vi "MIDI reader.vi"(8 "error in":errorcluster) -> (0 "error out":errorcluster, 2 "Note Events":T1[](array[typedef]), 3 "Array":T2(array[cluster]) {"U8" format="%x"; "Bytes" format="%02d"; "U8" format="%x"})   [LabVIEW 2016]
uses:
  Notes.ctl
  Midi data.ctl
panel:
  out "Time Sig Denom":u8
  out "data":u8[](array[numeric]) format="%x"
  out "Sequencer Event":string
  out "Device Name":string
  out "Program Name":string
  out "Cue Point":string
  out "Marker":string
  out "Lyric":string
  out "Instr Name":string
  out "CopyRight":string
  out "Text":string
  out "Track Name":string
  out "Key Signature":i8[](array[numeric])
  out "Time Sig":u8[](array[numeric])
  out "SMPTE Offset":u8[](array[numeric])
  out "MIDI Port":u8
  out "MIDI Channel":u8
  out "MIDI cue":u16
  out "size(s)":i32[](array[numeric])
  out "ms/b":u32
  out "Track length":u32
  out "Division":u16
  out "Number of tracks":u16
  out "Format":u16
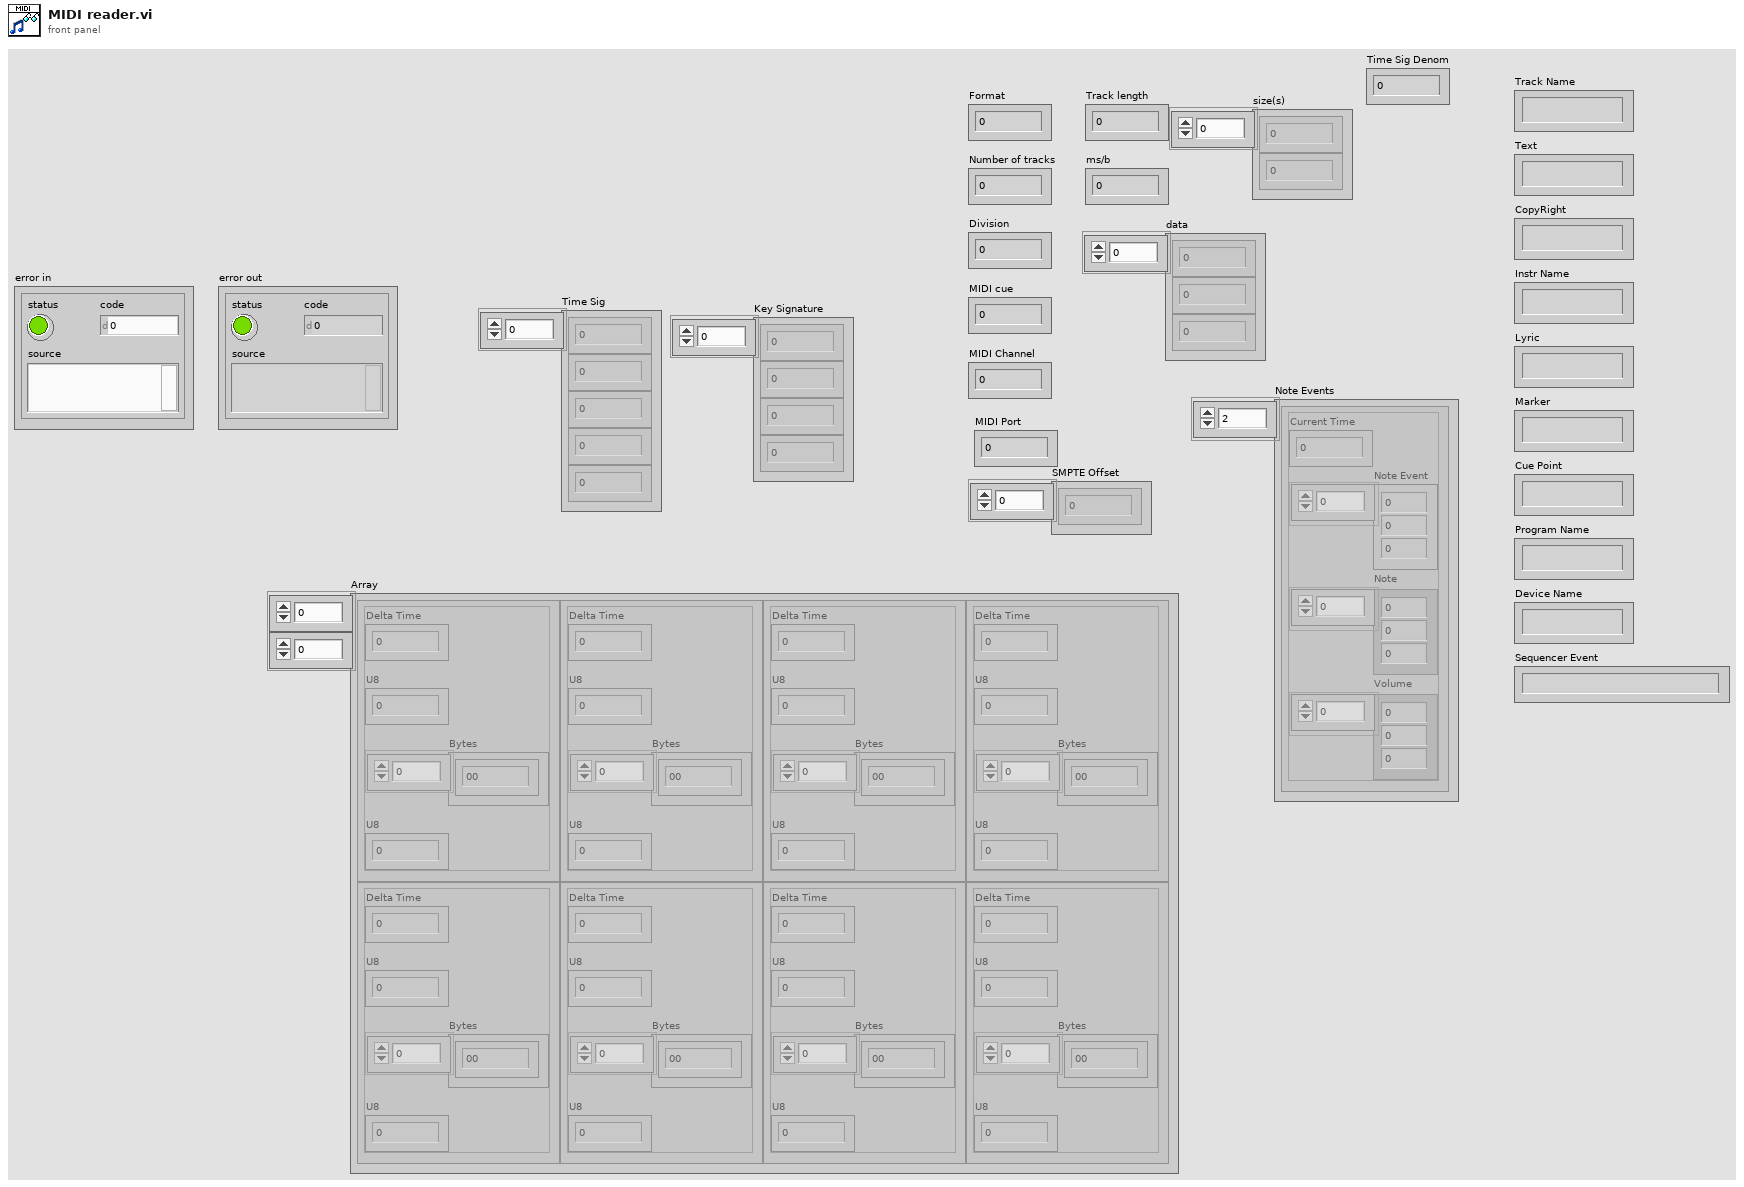
[diagram p1: front panel]
types:
  T1 = typedef "Notes.ctl" = cluster{"Current Time":u32, "Note Event":u32[], "Note":u32[], "Volume":u32[]}
  T2 = cluster{"Delta Time":u32, "U8":u8, "Bytes":u32[], "U8":u8}[][]
  T3 = enum16{"big-endian, network order", "native, host order", "little-endian"}
  T4 = cluster{"Delta Time":u32, "U8":u8, "Bytes":u32[], "U8":u8}[]
  T5 = typedef "Midi data.ctl" = cluster{"Delta Time":u32, "Event Status":u8, "Bytes":u32[], "Event Val":u8}
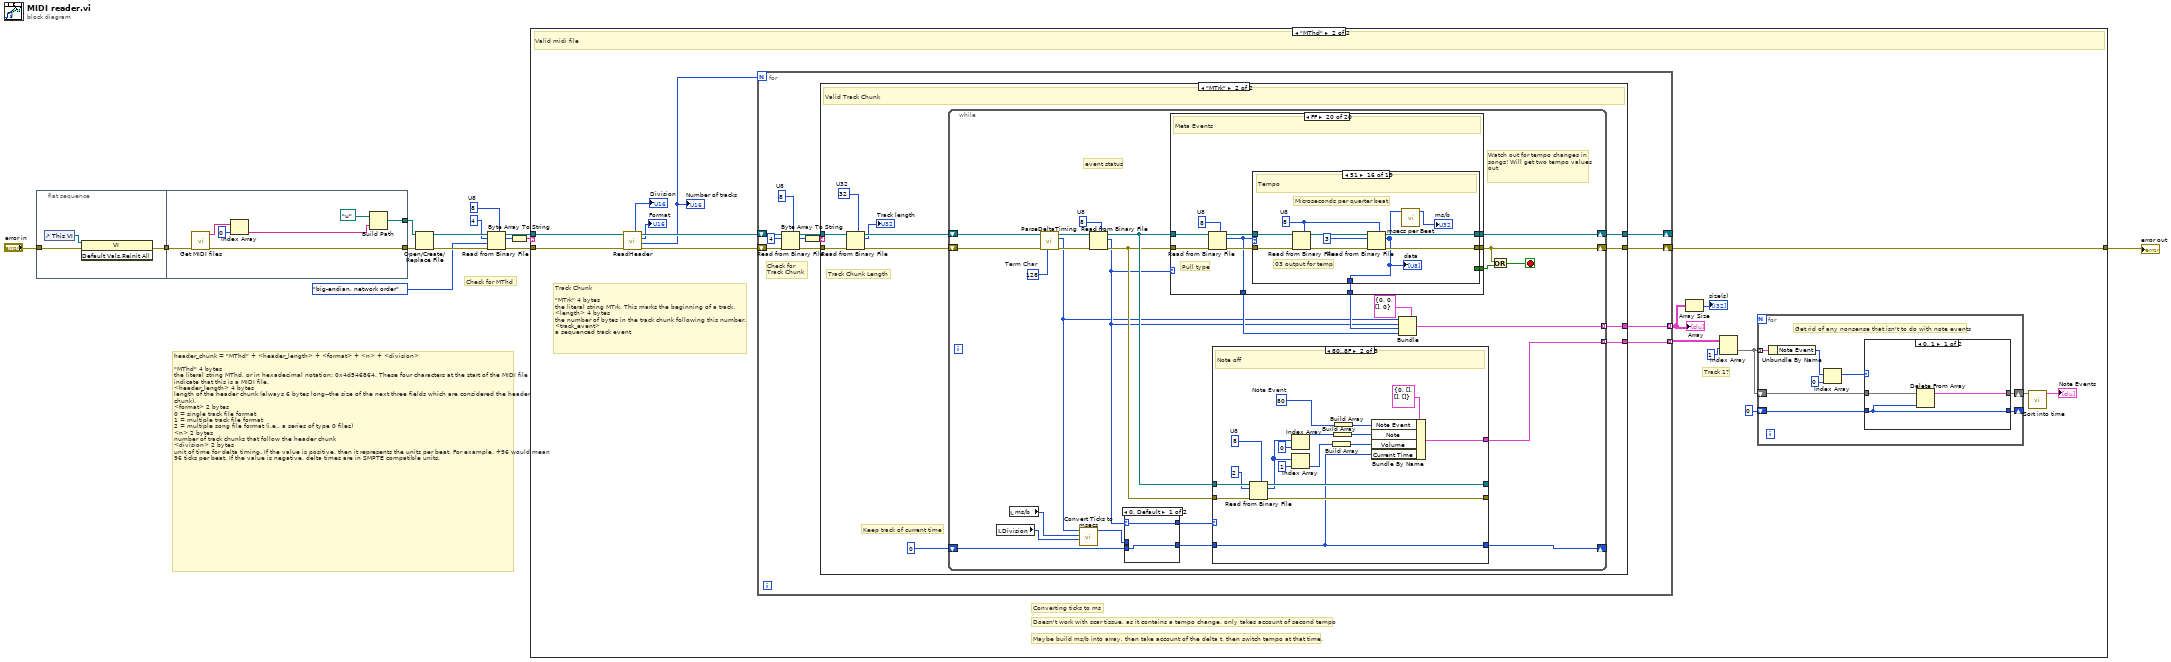
[diagram p0: block diagram]
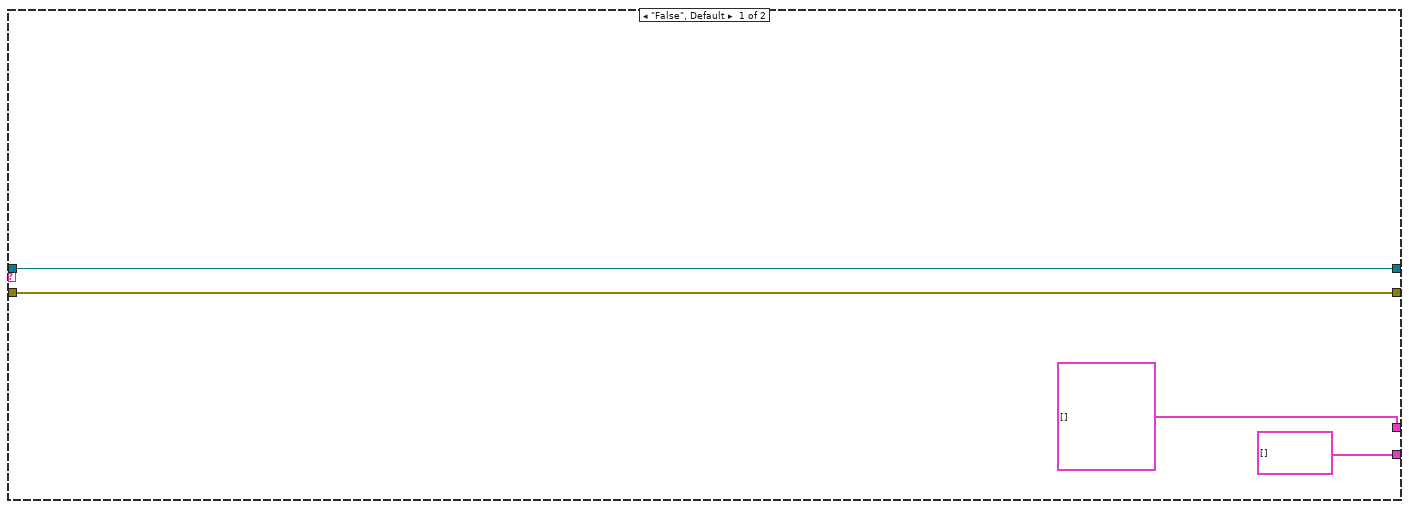
[diagram p3: hidden frame]
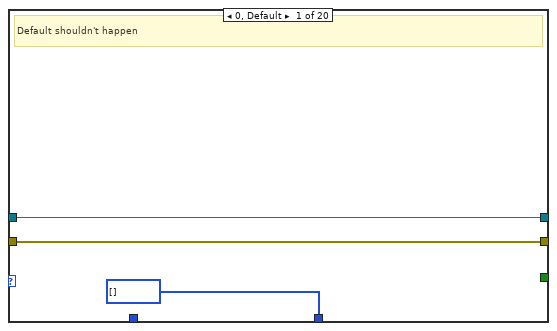
[diagram p4: hidden frame]
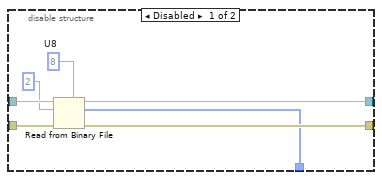
[diagram p6: hidden frame]
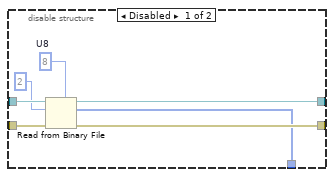
[diagram p8: hidden frame]
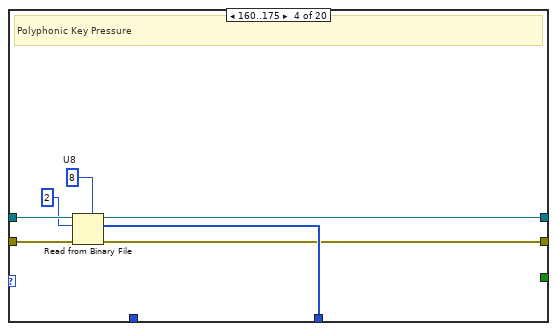
[diagram p9: hidden frame]
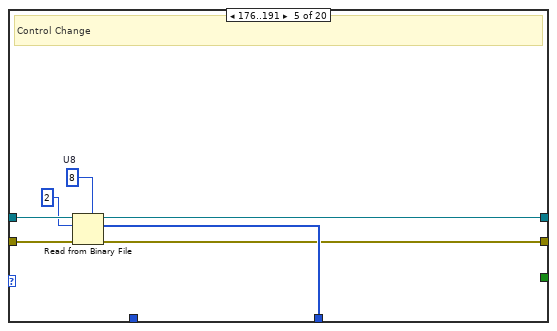
[diagram p10: hidden frame]
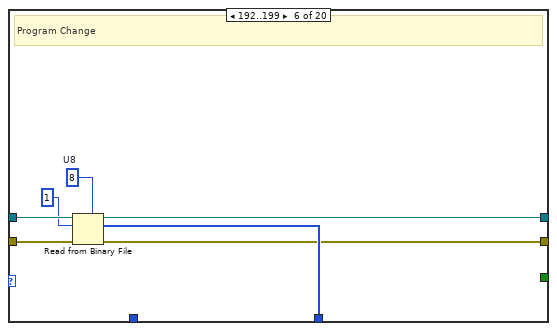
[diagram p11: hidden frame]
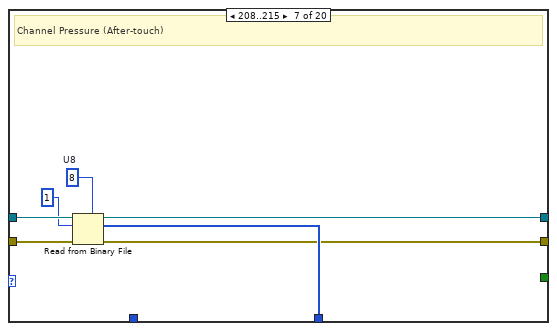
[diagram p12: hidden frame]
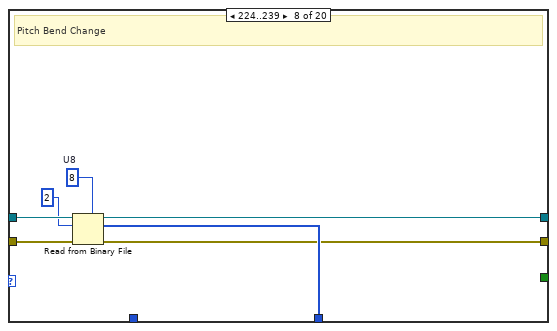
[diagram p13: hidden frame]
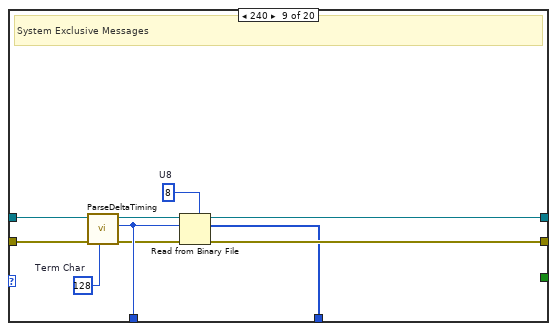
[diagram p14: hidden frame]
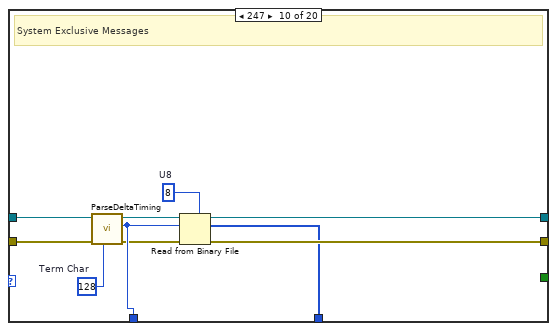
[diagram p15: hidden frame]
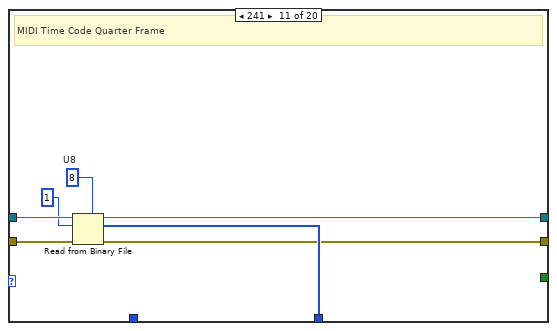
[diagram p16: hidden frame]
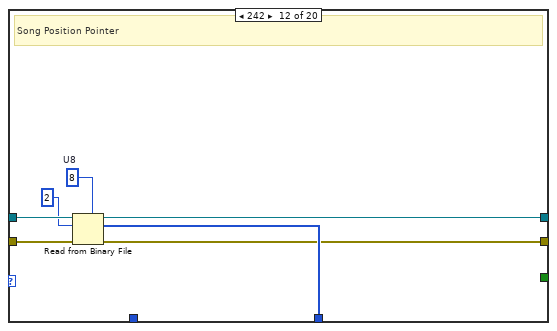
[diagram p17: hidden frame]
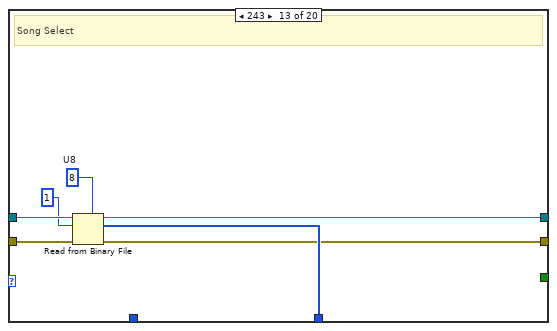
[diagram p18: hidden frame]
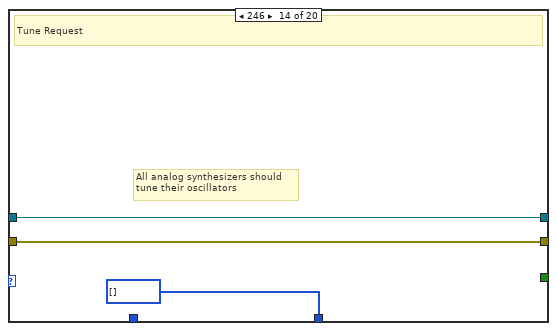
[diagram p19: hidden frame]
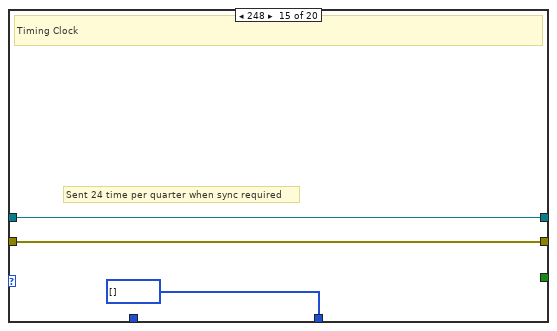
[diagram p20: hidden frame]
diagram:
  w10 = u8 8  # U8
  # "Check for MThd"
  # "header_chunk = \"MThd\" + <header_length> + <format> + <n> + <division>\n \n\"MThd\" 4 bytes\nthe literal string MThd, or in hexadecimal notation: 0x4d546864. These four characters at the start of the MIDI file indicate that this is a MIDI file.\n<header_length> 4 bytes\nlength of the header chunk (always 6 bytes long--the size of the next three fields which are considered the header chunk).\n<format> 2 bytes\n0 = single track file format \n1 = multiple track file format \n2 = multiple song file format (i.e., a series of type 0 files)\n<n> 2 bytes\nnumber of track chunks that follow the header chunk\n<division> 2 bytes\nunit of time for delta timing. If the value is positive, then it represents the units per beat. For example, +96 would mean 96 ticks per beat. If the value is negative, delta times are in SMPTE compatible units."
  n1 = flat-sequence {
    tunnel: [w16] -> w4
    tunnel: "error in" -> [w15]
    tunnel: [w23] -> w5
    tunnel: w4 -> [w24]
    tunnel: [w18] -> w1
    frame #0 {
      n2 = control-ref of="This VI"() -> (w17:refnum<vi>)
      n3 = invoke class="VI" method="Default Vals.Reinit All"(reference=w17, error in=w15) -> (error out=w16:errorcluster)  [unwired: 1 in, 2 out]
    }
    frame #1 {
      n4 = call "Get MIDI files.vi"("error in (no error)"=w24) -> ("error out"=w23:errorcluster, "Available MIDI Files"=w22:string[])  [unwired: 9 in]
      n5 = Index Array(array=w22, index=0) -> (element=w19:string)
      n6 = Build Path(base path=path "u:/" ("selected path"), name or relative path=w19) -> (appended path=w18:path)
    }
  }
  n7 = Open/Create/Replace File(file path (use dialog)=w1, error in=w5) -> (refnum out=w14:refnum<file>, error out=w13:errorcluster)  [unwired: 4 in, 1 out]
  n8 = Read from Binary File(5:w10, 8:w13, 9:T3."big-endian, network order" ("byte order (0:big-endian, network order)"), 10:4 ("count (1)"), 11:w14) -> (0:w6:errorcluster, 2:w9:u8[], 3:w7:refnum<file>)  [unwired: 1 in, 1 out]
  n9 = Byte Array To String(unsigned byte array=w9) -> (string=w8:string)
  n10 = case shown="\"MThd\"" w8 {
    tunnel: w7 -> [_ w41]
    tunnel: w6 -> [w25 w40]
    tunnel: [w25 w26] -> w3
    frame "False", Default {
      # "Not a midi file"
    }
    frame "MThd" {
      # "Track Chunk\n\n\"MTrk\" 4 bytes\nthe literal string MTrk. This marks the beginning of a track.\n<length> 4 bytes\nthe number of bytes in the track chunk following this number.\n<track_event>\na sequenced track event"
      # "Maybe build ms/b into array, then take account of the delta t, then switch tempo at that time."
      # "Doesn't work with scar tissue, as it contains a tempo change, only takes account of second tempo"
      # "Converting ticks to ms"
      # "Track 1?"
      # "Valid midi file"
      n11 = call "ReadHeader.vi"("error in (no error)"=w40, "Byte Stream File in"=w41) -> ("error out"=w38:errorcluster, "Number of tracks"=w35:u16, "Format"=→"Format":u16, "Byte Stream File out"=w39:refnum<file>, "Division"=→"Division":u16)  [unwired: 5 in]
      "Number of tracks" <- w35
      n12 = for {
        N: w35 -> [_]
        shift-right: [w45] -> _
        shift-left: w39 -> [w53]
        shift-right: [w44] -> w26
        shift-left: w38 -> [w52]
        tunnel: [w43] -> w33 mode=indexing
        tunnel: [w42] -> w32 mode=indexing
        w50 = u8 8  # U8
        # "Check for \nTrack Chunk"
        n13 = Read from Binary File(5:w50, 8:w52, 10:4 ("count (1)"), 11:w53) -> (0:w46:errorcluster, 2:w49:u8[], 3:w47:refnum<file>)  [unwired: 2 in, 1 out]
        n14 = Byte Array To String(unsigned byte array=w49) -> (string=w48:string)
        n15 = case shown="\"MTrk\"" w48 {
          tunnel: w47 -> [w57 w68]
          tunnel: w46 -> [w56 w67]
          tunnel: [w57 w63] -> w45
          tunnel: [w56 w62] -> w44
          tunnel: [T4 [] w61] -> w43
          tunnel: [T1[] [] w58] -> w42
          frame "False", Default {
          }
          frame "MTrk" {
            w66 = u32 32  # U32
            # "Keep track of current time"
            # "Track Chunk Length"
            # "Valid Track Chunk"
            n16 = Read from Binary File(5:w66, 8:w67, 11:w68) -> (0:w64:errorcluster, 2:→"Track length":u32, 3:w65:refnum<file>)  [unwired: 3 in, 1 out]
            n17 = while {
              tunnel: [w91] -> w61 mode=indexing
              shift-right: [w92] -> w63
              shift-left: w65 -> [w94]
              shift-right: [w82] -> w62
              shift-left: w64 -> [w93]
              tunnel: [w78] -> w58 mode=indexing
              shift-right: [w74] -> _
              shift-left: u32 0 ("Current Time") -> [w73]
              stop <- w81 stop-if-true
              w87 = 128  # Term Char
              w88 = u8 8  # U8
              # "Watch out for tempo changes in songs! Will get two tempo values out"
              # "event status"
              n18 = local read "Division"() -> (w69:u16)
              n19 = local read "ms/b"() -> (w70:u32)
              n20 = call "ParseDeltaTiming.vi"("TermChar (80h)"=w87, "error in (no error)"=w93, "Byte Stream File in"=w94) -> ("error out"=w90:errorcluster, "Delta Time"=w72:u32, "Byte Stream File out"=w89:refnum<file>)  [unwired: 6 in]
              n21 = call "Convert Ticks to msecs.vi"("Division"=w69, "ms/b"=w70, "Delta Time"=w72) -> ("Delta Time msec"=w71:u32)  [unwired: 8 in]
              n22 = Read from Binary File(5:w88, 8:w90, 11:w89) -> (0:w79:errorcluster, 2:w77:u8, 3:w80:refnum<file>)  [unwired: 3 in, 1 out]
              n23 = case shown="0, Default" w77 {
                selector: w77 -> [w421 w425]
                tunnel: [w421 w425] -> w76
                tunnel: w73 -> [w420 w424]
                tunnel: w71 -> [_ w423]
                tunnel: [w420 w422] -> w75
                frame 0, Default {
                }
                frame 128..159 {
                  n24 = Add(x=w423, y=w424) -> (x+y=w422:u32)
                }
              }
              n25 = case shown="FF" w77 {
                tunnel: w80 -> [w97 w102 w116 w132 w139 w146 w153 w160 w165 w175 w187 w194 w201 w204 w207 w210 w213 w216 w219 w225]
                tunnel: w79 -> [w96 w101 w115 w131 w138 w145 w152 w159 w164 w172 w186 w193 w200 w203 w206 w209 w212 w215 w218 w226]
                tunnel: [u8[] [] w98 w112 w128 w135 w142 w149 w156 w167 w177 w183 w190 w197 u8[] [] u8[] [] u8[] [] u8[] [] u8[] [] u8[] [] w221] -> w86
                tunnel: [w97 w100 w114 w127 w134 w141 w148 w155 w169 w179 w182 w189 w196 w204 w207 w210 w213 w216 w219 w229] -> w92
                tunnel: [w96 w99 w113 w126 w133 w140 w147 w154 w168 w178 w181 w188 w195 w203 w206 w209 w212 w215 w218 w228] -> w82
                tunnel: [_ _ _ _ _ _ _ _ _ _ _ _ _ _ _ _ _ _ _ w222] -> w83
                tunnel: [_ _ _ _ _ _ _ _ w163 w173 _ _ _ _ _ _ _ _ _ w220] -> w85
                frame 0, Default {
                  # "Default shouldn't happen"
                }
                frame 128..143 {
                  # "Note off"
                  n26 = disable-structure shown="Enabled" {
                    disable-tunnel: w102 -> [w109 w111]
                    disable-tunnel: w101 -> [w108 w110]
                    disable-tunnel: [w105 w111] -> w100
                    disable-tunnel: [w104 w110] -> w99
                    disable-tunnel: [w103 _] -> w98
                    frame Disabled {
                      w106 = u8 8  # U8
                      n27 = Read from Binary File(5:w106, 8:w108, 10:2 ("count (1)"), 11:w109) -> (0:w104:errorcluster, 2:w103:u8[], 3:w105:refnum<file>)  [unwired: 2 in, 1 out]
                    }
                    frame Enabled {
                    }
                  }
                }
                frame 144..159 {
                  # "Note On"
                  n28 = disable-structure shown="Enabled" {
                    disable-tunnel: w116 -> [w123 w125]
                    disable-tunnel: w115 -> [w122 w124]
                    disable-tunnel: [w119 w125] -> w114
                    disable-tunnel: [w118 w124] -> w113
                    disable-tunnel: [w117 _] -> w112
                    frame Disabled {
                      w120 = u8 8  # U8
                      n29 = Read from Binary File(5:w120, 8:w122, 10:2 ("count (1)"), 11:w123) -> (0:w118:errorcluster, 2:w117:u8[], 3:w119:refnum<file>)  [unwired: 2 in, 1 out]
                    }
                    frame Enabled {
                    }
                  }
                }
                frame 160..175 {
                  w129 = u8 8  # U8
                  # "Polyphonic Key Pressure"
                  n30 = Read from Binary File(5:w129, 8:w131, 10:2 ("count (1)"), 11:w132) -> (0:w126:errorcluster, 2:w128:u8[], 3:w127:refnum<file>)  [unwired: 2 in, 1 out]
                }
                frame 176..191 {
                  w136 = u8 8  # U8
                  # "Control Change"
                  n31 = Read from Binary File(5:w136, 8:w138, 10:2 ("count (1)"), 11:w139) -> (0:w133:errorcluster, 2:w135:u8[], 3:w134:refnum<file>)  [unwired: 2 in, 1 out]
                }
                frame 192..199 {
                  w143 = u8 8  # U8
                  # "Program Change"
                  n32 = Read from Binary File(5:w143, 8:w145, 10:1 ("count (1)"), 11:w146) -> (0:w140:errorcluster, 2:w142:u8[], 3:w141:refnum<file>)  [unwired: 2 in, 1 out]
                }
                frame 208..215 {
                  w150 = u8 8  # U8
                  # "Channel Pressure (After-touch)"
                  n33 = Read from Binary File(5:w150, 8:w152, 10:1 ("count (1)"), 11:w153) -> (0:w147:errorcluster, 2:w149:u8[], 3:w148:refnum<file>)  [unwired: 2 in, 1 out]
                }
                frame 224..239 {
                  w157 = u8 8  # U8
                  # "Pitch Bend Change"
                  n34 = Read from Binary File(5:w157, 8:w159, 10:2 ("count (1)"), 11:w160) -> (0:w154:errorcluster, 2:w156:u8[], 3:w155:refnum<file>)  [unwired: 2 in, 1 out]
                }
                frame 240 {
                  w161 = 128  # Term Char
                  w170 = u8 8  # U8
                  # "System Exclusive Messages"
                  n35 = call "ParseDeltaTiming.vi"("TermChar (80h)"=w161, "error in (no error)"=w164, "Byte Stream File in"=w165) -> ("error out"=w162:errorcluster, "Delta Time"=w163:u32, "Byte Stream File out"=w166:refnum<file>)  [unwired: 6 in]
                  n36 = Read from Binary File(5:w170, 8:w162, 10:w163, 11:w166) -> (0:w168:errorcluster, 2:w167:u8[], 3:w169:refnum<file>)  [unwired: 2 in, 1 out]
                }
                frame 247 {
                  w176 = 128  # Term Char
                  w180 = u8 8  # U8
                  # "System Exclusive Messages"
                  n37 = call "ParseDeltaTiming.vi"("TermChar (80h)"=w176, "error in (no error)"=w172, "Byte Stream File in"=w175) -> ("error out"=w171:errorcluster, "Delta Time"=w173:u32, "Byte Stream File out"=w174:refnum<file>)  [unwired: 6 in]
                  n38 = Read from Binary File(5:w180, 8:w171, 10:w173, 11:w174) -> (0:w178:errorcluster, 2:w177:u8[], 3:w179:refnum<file>)  [unwired: 2 in, 1 out]
                }
                frame 241 {
                  w184 = u8 8  # U8
                  # "MIDI Time Code Quarter Frame"
                  n39 = Read from Binary File(5:w184, 8:w186, 10:1 ("count (1)"), 11:w187) -> (0:w181:errorcluster, 2:w183:u8[], 3:w182:refnum<file>)  [unwired: 2 in, 1 out]
                }
                frame 242 {
                  w191 = u8 8  # U8
                  # "Song Position Pointer"
                  n40 = Read from Binary File(5:w191, 8:w193, 10:2 ("count (1)"), 11:w194) -> (0:w188:errorcluster, 2:w190:u8[], 3:w189:refnum<file>)  [unwired: 2 in, 1 out]
                }
                frame 243 {
                  w198 = u8 8  # U8
                  # "Song Select"
                  n41 = Read from Binary File(5:w198, 8:w200, 10:1 ("count (1)"), 11:w201) -> (0:w195:errorcluster, 2:w197:u8[], 3:w196:refnum<file>)  [unwired: 2 in, 1 out]
                }
                frame 246 {
                  # "All analog synthesizers should \ntune their oscillators"
                  # "Tune Request"
                }
                frame 248 {
                  # "Sent 24 time per quarter when sync required"
                  # "Timing Clock"
                }
                frame 250 {
                  # "Starts current sequence playing"
                  # "Start"
                }
                frame 251 {
                  # "Continue sequence"
                }
                frame 252 {
                  # "Stop sequence"
                }
                frame 254 {
                  # "Active Sensing"
                }
                frame 255 {
                  w227 = u8 8  # U8
                  # "Pull type"
                  # "Meta Events"
                  n42 = Read from Binary File(5:w227, 8:w226, 11:w225) -> (0:w223:errorcluster, 2:w220:u8, 3:w224:refnum<file>)  [unwired: 3 in, 1 out]
                  n43 = case shown="51" w220 {
                    tunnel: [w232 w236 w245 w256 w267 w278 w289 w300 w311 w322 w333 w344 w358 w367 w376 w385 w394 w405 w415] -> w229
                    tunnel: [w231 w235 w244 w255 w266 w277 w288 w299 w310 w321 w332 w343 w357 w366 w375 w384 w393 w404 w414] -> w228
                    tunnel: w224 -> [w232 w241 w253 w264 w275 w286 w297 w308 w319 w330 w341 w352 w362 w371 w377 w389 w398 w409 w419]
                    tunnel: w223 -> [w231 w242 w252 w263 w274 w285 w296 w307 w318 w329 w340 w351 w361 w370 w374 w388 w397 w408 w418]
                    tunnel: [_ _ _ _ _ _ _ _ _ _ _ _ _ _ TRUE _ _ _ _] -> w222
                    tunnel: [u32[] [] w233 w247 w258 w269 w280 w291 w302 w313 w324 w335 w346 w354 w363 w372 w381 w390 w401 w411] -> w221
                    frame 255, Default {
                    }
                    frame 0 {
                      w237 = u16 16  # U16
                      w240 = u8 8  # U8
                      # "02"
                      # "Sequence number"
                      n44 = Read from Binary File(5:w240, 8:w242, 10:1 ("count (1)"), 11:w241) -> (0:w239:errorcluster, 3:w238:refnum<file>)  [unwired: 2 in, 2 out]
                      n45 = Read from Binary File(5:w237, 8:w239, 11:w238) -> (0:w235:errorcluster, 2:w234:u16, 3:w236:refnum<file>)  [unwired: 3 in, 1 out]
                      "MIDI cue" <- w234
                      n46 = Build Array(w234) -> (w233:u16[])
                    }
                    frame 3 {
                      w248 = u8 8  # U8
                      w254 = 128  # Term Char
                      # "Sequence/Track Name"
                      n47 = call "ParseDeltaTiming.vi"("TermChar (80h)"=w254, "error in (no error)"=w252, "Byte Stream File in"=w253) -> ("error out"=w251:errorcluster, "Delta Time"=w249:u32, "Byte Stream File out"=w250:refnum<file>)  [unwired: 6 in]
                      n48 = Read from Binary File(5:w248, 8:w251, 10:w249, 11:w250) -> (0:w244:errorcluster, 2:w247:u8[], 3:w245:refnum<file>)  [unwired: 2 in, 1 out]
                      n49 = Byte Array To String(unsigned byte array=w247) -> (string=→"Track Name":string)
                    }
                    frame 1 {
                      w259 = u8 8  # U8
                      w265 = 128  # Term Char
                      # "Text"
                      n50 = call "ParseDeltaTiming.vi"("TermChar (80h)"=w265, "error in (no error)"=w263, "Byte Stream File in"=w264) -> ("error out"=w262:errorcluster, "Delta Time"=w260:u32, "Byte Stream File out"=w261:refnum<file>)  [unwired: 6 in]
                      n51 = Read from Binary File(5:w259, 8:w262, 10:w260, 11:w261) -> (0:w255:errorcluster, 2:w258:u8[], 3:w256:refnum<file>)  [unwired: 2 in, 1 out]
                      n52 = Byte Array To String(unsigned byte array=w258) -> (string=→"Text":string)
                    }
                    frame 2 {
                      w270 = u8 8  # U8
                      w276 = 128  # Term Char
                      # "copyright"
                      n53 = call "ParseDeltaTiming.vi"("TermChar (80h)"=w276, "error in (no error)"=w274, "Byte Stream File in"=w275) -> ("error out"=w273:errorcluster, "Delta Time"=w271:u32, "Byte Stream File out"=w272:refnum<file>)  [unwired: 6 in]
                      n54 = Read from Binary File(5:w270, 8:w273, 10:w271, 11:w272) -> (0:w266:errorcluster, 2:w269:u8[], 3:w267:refnum<file>)  [unwired: 2 in, 1 out]
                      n55 = Byte Array To String(unsigned byte array=w269) -> (string=→"CopyRight":string)
                    }
                    frame 4 {
                      w281 = u8 8  # U8
                      w287 = 128  # Term Char
                      # "Instrument Name"
                      n56 = call "ParseDeltaTiming.vi"("TermChar (80h)"=w287, "error in (no error)"=w285, "Byte Stream File in"=w286) -> ("error out"=w284:errorcluster, "Delta Time"=w282:u32, "Byte Stream File out"=w283:refnum<file>)  [unwired: 6 in]
                      n57 = Read from Binary File(5:w281, 8:w284, 10:w282, 11:w283) -> (0:w277:errorcluster, 2:w280:u8[], 3:w278:refnum<file>)  [unwired: 2 in, 1 out]
                      n58 = Byte Array To String(unsigned byte array=w280) -> (string=→"Instr Name":string)
                    }
                    frame 5 {
                      w292 = u8 8  # U8
                      w298 = 128  # Term Char
                      # "Lyric"
                      n59 = call "ParseDeltaTiming.vi"("TermChar (80h)"=w298, "error in (no error)"=w296, "Byte Stream File in"=w297) -> ("error out"=w295:errorcluster, "Delta Time"=w293:u32, "Byte Stream File out"=w294:refnum<file>)  [unwired: 6 in]
                      n60 = Read from Binary File(5:w292, 8:w295, 10:w293, 11:w294) -> (0:w288:errorcluster, 2:w291:u8[], 3:w289:refnum<file>)  [unwired: 2 in, 1 out]
                      n61 = Byte Array To String(unsigned byte array=w291) -> (string=→"Lyric":string)
                    }
                    frame 6 {
                      w303 = u8 8  # U8
                      w309 = 128  # Term Char
                      # "Marker"
                      n62 = call "ParseDeltaTiming.vi"("TermChar (80h)"=w309, "error in (no error)"=w307, "Byte Stream File in"=w308) -> ("error out"=w306:errorcluster, "Delta Time"=w304:u32, "Byte Stream File out"=w305:refnum<file>)  [unwired: 6 in]
                      n63 = Read from Binary File(5:w303, 8:w306, 10:w304, 11:w305) -> (0:w299:errorcluster, 2:w302:u8[], 3:w300:refnum<file>)  [unwired: 2 in, 1 out]
                      n64 = Byte Array To String(unsigned byte array=w302) -> (string=→"Marker":string)
                    }
                    frame 7 {
                      w314 = u8 8  # U8
                      w320 = 128  # Term Char
                      # "Cue Point"
                      n65 = call "ParseDeltaTiming.vi"("TermChar (80h)"=w320, "error in (no error)"=w318, "Byte Stream File in"=w319) -> ("error out"=w317:errorcluster, "Delta Time"=w315:u32, "Byte Stream File out"=w316:refnum<file>)  [unwired: 6 in]
                      n66 = Read from Binary File(5:w314, 8:w317, 10:w315, 11:w316) -> (0:w310:errorcluster, 2:w313:u8[], 3:w311:refnum<file>)  [unwired: 2 in, 1 out]
                      n67 = Byte Array To String(unsigned byte array=w313) -> (string=→"Cue Point":string)
                    }
                    frame 8 {
                      w325 = u8 8  # U8
                      w331 = 128  # Term Char
                      # "Program Name"
                      n68 = call "ParseDeltaTiming.vi"("TermChar (80h)"=w331, "error in (no error)"=w329, "Byte Stream File in"=w330) -> ("error out"=w328:errorcluster, "Delta Time"=w326:u32, "Byte Stream File out"=w327:refnum<file>)  [unwired: 6 in]
                      n69 = Read from Binary File(5:w325, 8:w328, 10:w326, 11:w327) -> (0:w321:errorcluster, 2:w324:u8[], 3:w322:refnum<file>)  [unwired: 2 in, 1 out]
                      n70 = Byte Array To String(unsigned byte array=w324) -> (string=→"Program Name":string)
                    }
                    frame 9 {
                      w336 = u8 8  # U8
                      w342 = 128  # Term Char
                      # "Device Name"
                      n71 = call "ParseDeltaTiming.vi"("TermChar (80h)"=w342, "error in (no error)"=w340, "Byte Stream File in"=w341) -> ("error out"=w339:errorcluster, "Delta Time"=w337:u32, "Byte Stream File out"=w338:refnum<file>)  [unwired: 6 in]
                      n72 = Read from Binary File(5:w336, 8:w339, 10:w337, 11:w338) -> (0:w332:errorcluster, 2:w335:u8[], 3:w333:refnum<file>)  [unwired: 2 in, 1 out]
                      n73 = Byte Array To String(unsigned byte array=w335) -> (string=→"Device Name":string)
                    }
                    frame 127 {
                      w347 = u8 8  # U8
                      w353 = 128  # Term Char
                      # "Sequencer Specific Event"
                      n74 = call "ParseDeltaTiming.vi"("TermChar (80h)"=w353, "error in (no error)"=w351, "Byte Stream File in"=w352) -> ("error out"=w350:errorcluster, "Delta Time"=w348:u32, "Byte Stream File out"=w349:refnum<file>)  [unwired: 6 in]
                      n75 = Read from Binary File(5:w347, 8:w350, 10:w348, 11:w349) -> (0:w343:errorcluster, 2:w346:u8[], 3:w344:refnum<file>)  [unwired: 2 in, 1 out]
                      n76 = Byte Array To String(unsigned byte array=w346) -> (string=→"Sequencer Event":string)
                    }
                    frame 32 {
                      w356 = u8 8  # U8
                      # "0-15"
                      # "01"
                      # "MIDI Channel Prefix"
                      n77 = Read from Binary File(5:w356, 8:w361, 11:w362) -> (0:w360:errorcluster, 3:w359:refnum<file>)  [unwired: 3 in, 2 out]
                      n78 = Read from Binary File(5:w356, 8:w360, 11:w359) -> (0:w357:errorcluster, 2:w355:u8, 3:w358:refnum<file>)  [unwired: 3 in, 1 out]
                      "MIDI Channel" <- w355
                      n79 = Build Array(w355) -> (w354:u8[])
                    }
                    frame 33 {
                      w365 = u8 8  # U8
                      # "0-127"
                      # "01"
                      # "MIDI Port"
                      n80 = Read from Binary File(5:w365, 8:w370, 11:w371) -> (0:w369:errorcluster, 3:w368:refnum<file>)  [unwired: 3 in, 2 out]
                      n81 = Read from Binary File(5:w365, 8:w369, 11:w368) -> (0:w366:errorcluster, 2:w364:u8, 3:w367:refnum<file>)  [unwired: 3 in, 1 out]
                      "MIDI Port" <- w364
                      n82 = Build Array(w364) -> (w363:u8[])
                    }
                    frame 47 {
                      w379 = u8 8  # U8
                      # "End of Track"
                      n83 = Read from Binary File(5:w379, 8:w374, 10:1 ("count (1)"), 11:w377) -> (0:w375:errorcluster, 2:w372:u8[], 3:w376:refnum<file>)  [unwired: 2 in, 1 out]
                    }
                    frame 81 {
                      w382 = u8 8  # U8
                      # "Microseconds per quarter beat"
                      # "03 output for temp"
                      # "Tempo"
                      n84 = Read from Binary File(5:w382, 8:w388, 11:w389) -> (0:w387:errorcluster, 3:w386:refnum<file>)  [unwired: 3 in, 2 out]
                      n85 = Read from Binary File(5:w382, 8:w387, 10:3 ("count (1)"), 11:w386) -> (0:w384:errorcluster, 2:w381:u8[], 3:w385:refnum<file>)  [unwired: 2 in, 1 out]
                      "data" <- w381
                      n86 = call "msecs per Beat.vi"("tt tt tt"=w381) -> ("ms per beat"=→"ms/b":u32)  [unwired: 10 in]
                    }
                    frame 84 {
                      w391 = u8 8  # U8
                      # "05"
                      # "SMPTE Offset"
                      n87 = Read from Binary File(5:w391, 8:w397, 11:w398) -> (0:w396:errorcluster, 3:w395:refnum<file>)  [unwired: 3 in, 2 out]
                      n88 = Read from Binary File(5:w391, 8:w396, 10:5 ("count (1)"), 11:w395) -> (0:w393:errorcluster, 2:w390:u8[], 3:w394:refnum<file>)  [unwired: 2 in, 1 out]
                      "SMPTE Offset" <- w390
                    }
                    frame 88 {
                      w402 = u8 8  # U8
                      # "04"
                      # "Time Signature"
                      n89 = Read from Binary File(5:w402, 8:w408, 11:w409) -> (0:w407:errorcluster, 3:w406:refnum<file>)  [unwired: 3 in, 2 out]
                      n90 = Read from Binary File(5:w402, 8:w407, 10:4 ("count (1)"), 11:w406) -> (0:w404:errorcluster, 2:w401:u8[], 3:w405:refnum<file>)  [unwired: 2 in, 1 out]
                      "Time Sig" <- w401
                      n91 = Index Array(array=w401, index=1) -> (element=→"Time Sig Denom":u8)
                    }
                    frame 89 {
                      w410 = i8 8  # U8
                      w412 = u8 8  # U8
                      # "02"
                      # "Key Signature"
                      n92 = Read from Binary File(5:w412, 8:w418, 11:w419) -> (0:w417:errorcluster, 3:w416:refnum<file>)  [unwired: 3 in, 2 out]
                      n93 = Read from Binary File(5:w410, 8:w417, 10:2 ("count (1)"), 11:w416) -> (0:w414:errorcluster, 2:w411:i8[], 3:w415:refnum<file>)  [unwired: 2 in, 1 out]
                      "Key Signature" <- w411
                    }
                  }
                }
              }
              n94 = case shown="80..8F" w76 {
                tunnel: w80 -> [w429 w447 w465]
                tunnel: w79 -> [w428 w446 w464]
                tunnel: [w429 w443 w461] -> _
                tunnel: [w428 w442 w460] -> _
                tunnel: [T1 {"Current Time"=0, "Note Event"=[], "Note"=[], "Volume"=[]} ("Cluster") w441 w453] -> w78
                tunnel: w75 -> [w427 w439 w454]
                tunnel: [w427 w439 w454] -> w74
                frame 0, Default {
                  # "Any event that isn't a note on/off"
                }
                frame 128..143 {
                  w440 = u8 80  # Note Event
                  w444 = u8 8  # U8
                  # "Note off"
                  n95 = Read from Binary File(5:w444, 8:w446, 10:2 ("count (1)"), 11:w447) -> (0:w442:errorcluster, 2:w436:u8[], 3:w443:refnum<file>)  [unwired: 2 in, 1 out]
                  n96 = Index Array(array=w436, index=0) -> (element=w438:u8)
                  n97 = Index Array(array=w436, index=1) -> (element=w434:u8)
                  n98 = Build Array(w434) -> (w431:u8[])
                  n99 = Build Array(w438) -> (w432:u8[])
                  n100 = Build Array(w440) -> (w430:u8[])
                  n101 = Bundle By Name(cluster=T1 {"Current Time"=0, "Note Event"=[], "Note"=[], "Volume"=[]} ("Array"), "Note Event"=w430, "Note"=w432, "Volume"=w431, "Current Time"=w439) -> (w441:T1)
                }
                frame 144..159 {
                  w459 = u8 90  # Note Event
                  w462 = u8 8  # U8
                  # "Note On"
                  n102 = Read from Binary File(5:w462, 8:w464, 10:2 ("count (1)"), 11:w465) -> (0:w460:errorcluster, 2:w455:u8[], 3:w461:refnum<file>)  [unwired: 2 in, 1 out]
                  n103 = Index Array(array=w455, index=0) -> (element=w451:u8)
                  n104 = Index Array(array=w455, index=1) -> (element=w456:u8)
                  n105 = Build Array(w459) -> (w448:u8[])
                  n106 = Build Array(w456) -> (w449:u8[])
                  n107 = Build Array(w451) -> (w450:u8[])
                  n108 = Bundle By Name(cluster=T1 {"Current Time"=0, "Note Event"=[], "Note"=[], "Volume"=[]} ("Array"), "Note Event"=w448, "Note"=w450, "Volume"=w449, "Current Time"=w454) -> (w453:T1)
                }
              }
              n109 = Bundle(cluster=T5 {"Delta Time"=0, "Event Status"=0, "Bytes"=[], "Event Val"=0} ("output cluster"), "Delta Time"=w72, "Event Status"=w77, "Bytes"=w86, "Event Val"=w85) -> (w91:T5)
              n110 = Or(x=w82, y=w83) -> (x .or. y?=w81:bool)
            }
          }
        }
      }
      "Array" <- w33
      n111 = Array Size(array=w33) -> (size(s)=→"size(s)":i32[])
      n112 = Index Array(array=w32, index (row)=1) -> (element=w31:T1[])  [unwired: 1 in]
      n113 = for {
        tunnel: w31 -> [w472] mode=indexing
        shift-right: [w469] -> w28
        shift-left: w31 -> [w471]
        shift-right: [w468] -> _
        shift-left: 0 -> [w470]
        # "Get rid of any nonsense that isn't to do with note events"
        n114 = Unbundle By Name(w472) -> ("Note Event"=w473:u32[])
        n115 = Index Array(array=w473, index=0) -> (element=w467:u32)
        n116 = case shown="0, 1" w467 {
          tunnel: w471 -> [w476 w479]
          tunnel: [w475 w479] -> w469
          tunnel: w470 -> [w474 w478]
          tunnel: [w474 w477] -> w468
          frame 0, 1 {
            n117 = Delete From Array(array=w476, index=w474) -> (array with subset deleted=w475:T1[])  [unwired: 1 in, 1 out]
          }
          frame Default {
            n118 = Increment(x=w478) -> (x+1=w477:i32)
          }
        }
      }
      n119 = call "Sort into time.vi"("Note Events in"=w28) -> ("Note Events out"=→"Note Events":T1[])  [unwired: 10 in]
    }
  }
  "error out" <- w3
